vi "binary_to_timestamp.vi"(0 "binaryTimestampWithOffset":u8[](array[numeric])) -> (1 "timestamp":dbl, 2 "offset":dbl)   [LabVIEW 2020]
panel:
  out "(hi.lo)":u64
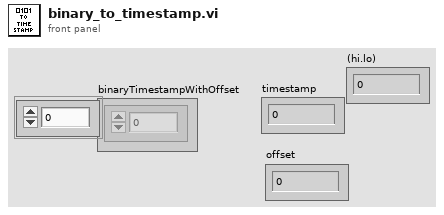
[diagram p1: front panel]
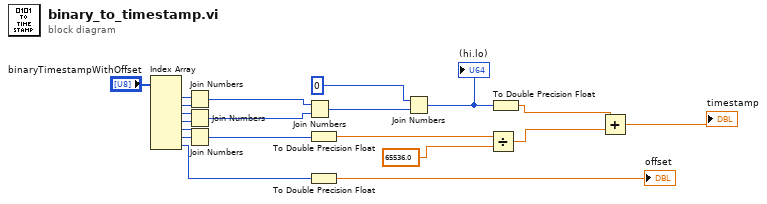
[diagram p0: block diagram]
diagram:
  n1 = Index Array(array="binaryTimestampWithOffset") -> (element #1=w5:u8, element #2=w6:u8, element #3=w7:u8, element #4=w8:u8, element #5=w9:u8, element #6=w10:u8, element #7=w3:u8)  [unwired: 7 in]
  n2 = Join Numbers(hi=w5, lo=w6) -> ((hi.lo)=w11:u16)
  n3 = Join Numbers(hi=w7, lo=w8) -> ((hi.lo)=w12:u16)
  n4 = Join Numbers(hi=w9, lo=w10) -> ((hi.lo)=w16:u16)
  n5 = Join Numbers(hi=w11, lo=w12) -> ((hi.lo)=w13:u32)
  n6 = To Double Precision Float(number=w16) -> (double precision float=w17:dbl)
  n7 = To Double Precision Float(number=w3) -> (double precision float=→"offset":dbl)
  n8 = Join Numbers(hi=u32 0, lo=w13) -> ((hi.lo)=w15:u64)
  "(hi.lo)" <- w15
  n9 = Divide(x=w17, y=65536.0) -> (x/y=w20:dbl)
  n10 = To Double Precision Float(number=w15) -> (double precision float=w19:dbl)
  n11 = Add(x=w19, y=w20) -> (x+y=→"timestamp":dbl)
